vi "Global_Read_INI_Sub_VI.vi"(0 "Config File Path":path) -> (4 "output cluster":T1)   [LabVIEW 2017]
uses:
  <vilib>/Utility/config.llb/Read Key (String).vi
  <vilib>/Utility/config.llb/Read Key (U32).vi
  <vilib>/Utility/config.llb/Read Key (Path).vi
  <vilib>/Utility/config.llb/NI_LVConfig.lvlib
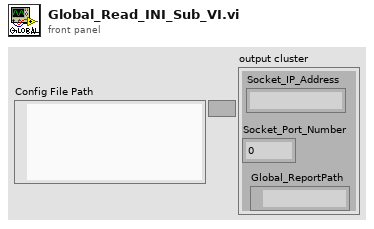
[diagram p1: front panel]
types:
  T1 = cluster{"Socket_IP_Address":string, "Socket_Port_Number":u16, "Global_ReportPath":path}
  T2 = typedef "NI_LVConfig.lvlib/Config Data RefNum.ctl" = refnum<k1>
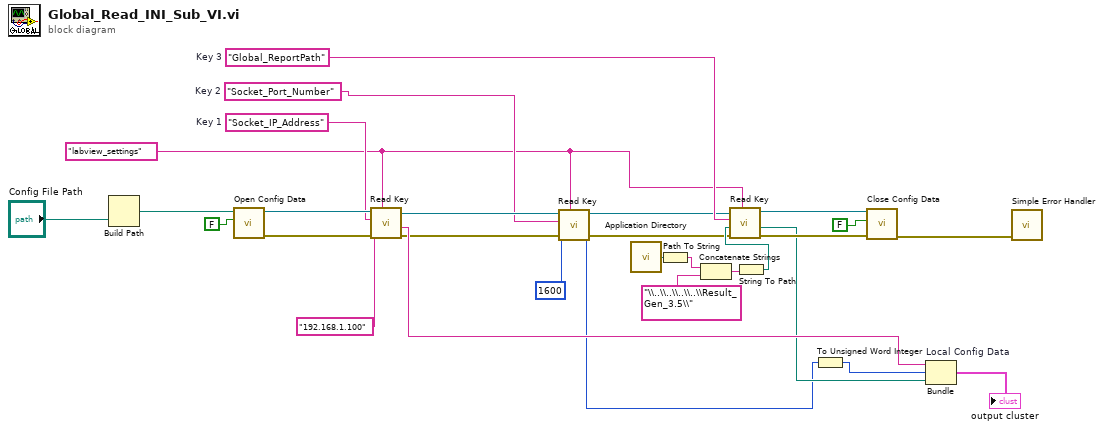
[diagram p0: block diagram]
diagram:
  w14 = "Global_ReportPath"  # Key 3
  w5 = "Socket_Port_Number"  # Key 2
  w10 = "Socket_IP_Address"  # Key 1
  w4 = "labview_settings" ("section")
  n1 = Build Path(name or relative path="Config File Path") -> (appended path=w21:path)  [unwired: 1 in]
  n2 = call <vilib>:"Open Config Data.vi"("create file if necessary (T)"=FALSE ("create file if necessary? (T)"), "configuration file path"=w21) -> ("error out"=w12:errorcluster, "refnum"=w13:T2)  [unwired: 7 in, 1 out]
  n3 = call-poly <vilib>:"Read Key.vi"("section"=w4, "error in (no error)"=w12, "default value"="192.168.1.100", "key"=w10, "refnum"=w13) -> ("error out"=w9:errorcluster, "value"=w24:string, "refnum out"=w6:T2)  [unwired: 1 in, 3 out]
  n4 = call-poly <vilib>:"Read Key.vi"("section"=w4, "error in (no error)"=w9, "default value"=u32 1600, "key"=w5, "refnum"=w6) -> ("error out"=w8:errorcluster, "value"=w2:u32, "refnum out"=w7:T2)  [unwired: 4 out]
  n5 = call <vilib>:"Application Directory.vi"() -> ("Application Directory"=w17:path)
  n6 = Path To String(path=w17) -> (string=w20:string)
  n7 = Concatenate Strings(w20, "\\..\\..\\..\\..\\Result_Gen_3.5\\" ("string")) -> (w18:string)
  n8 = String To Path(string=w18) -> (path=w16:path)
  n9 = call-poly <vilib>:"Read Key.vi"("section"=w4, "error in (no error)"=w8, "default value"=w16, "key"=w14, "refnum"=w7) -> ("error out"=w25:errorcluster, "value"=w15:path, "refnum out"=w26:T2)  [unwired: 1 in, 3 out]
  n10 = To Unsigned Word Integer(number=w2) -> (unsigned 16bit integer=w23:u16)
  n11 = call <vilib>:"Close Config Data.vi"("error in (no error)"=w25, "write file if changed (T)"=FALSE ("write configuration file? (T)"), "refnum"=w26) -> ("error out"=w29:errorcluster)  [unwired: 8 out]
  n12 = Bundle "Local Config Data"("value"=w24, w23, "value"=w15) -> (→"output cluster":cluster{"value":string, u16, "value":path})  [unwired: 1 in]
  n13 = call <vilib>:"Simple Error Handler.vi"("error in (no error)"=w29) -> ()  [unwired: 1 in, 8 out]
